vi "translate.vi"(0 "reference":refnum<class "PointNode.lvclass">, 1 "dx":dbl format="%.2f", 2 "dy":dbl format="%.2f", 5 "error in (no error)":errorcluster) -> (14 "reference out":refnum<class "PointNode.lvclass">, 19 "error out":errorcluster)   [LabVIEW 2016, in "PointNode.lvclass"]
doc: "public void translate(double dx, double dy)"
uses:
  <resource>/Framework/Providers/Open_GDS/UML/PointNode_class/PointNode.lvclass
  C:/Program Files (x86)/National Instruments/LabVIEW 2016/resource/Framework/Providers/Open_GDS/UML/AbstractNode_class/AbstractNode.lvclass
  <resource>/Framework/Providers/Open_GDS/UML/General/Point/Point Point2D.ctl
  <resource>/Framework/Providers/Open_GDS/UML/AbstractNode_class/AbstractNode.lvclass
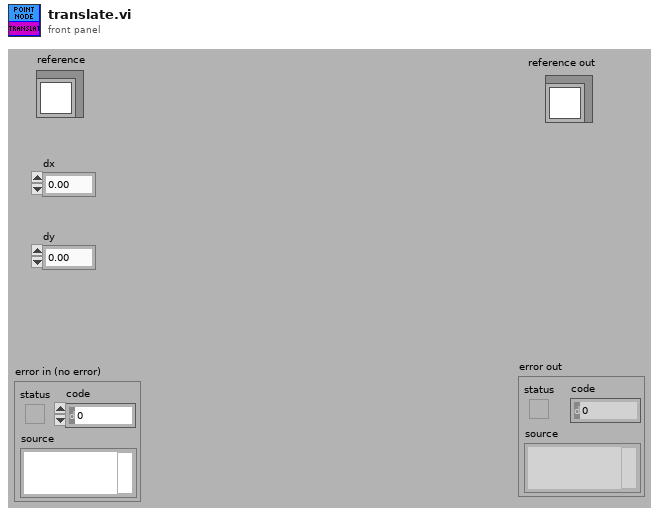
[diagram p1: front panel]
types:
  T1 = typedef "Point Point2D.ctl" = cluster{"x":dbl, "y":dbl}
  T2 = typedef "PointNode.lvclass/ObjectAttributes.ctl" = cluster{"point":T1}
  T3 = typedef "AbstractNode.lvclass/ObjectAttributes.ctl" = cluster{"parent":refnum<class "AbstractNode.lvclass">, "children":refnum<class "AbstractNode.lvclass">[], "Hidden":bool}
  T4 = typedef "Rectangle Rectangle2D.ctl" = cluster{"x":dbl, "y":dbl, "width":dbl, "height":dbl}
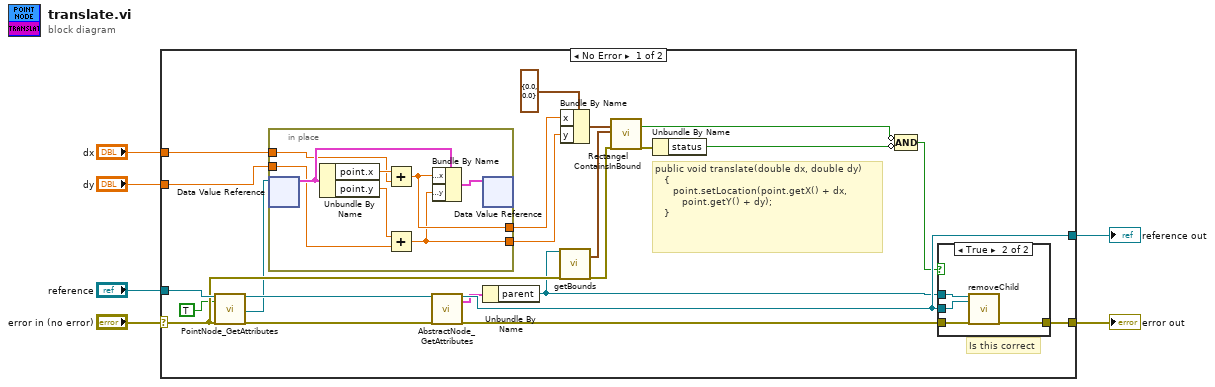
[diagram p0: block diagram]
diagram:
  n1 = case shown="No Error" "error in (no error)" {
    selector: "error in (no error)" -> [w24 w43]
    tunnel: "reference" -> [w29 w44]
    tunnel: [w28 w43] -> w5
    tunnel: [w27 w44] -> w4
    tunnel: "dx" -> [w12 _]
    tunnel: "dy" -> [w11 _]
    frame No Error {
      # "Is this correct"
      # "public void translate(double dx, double dy)\n   {\n      point.setLocation(point.getX() + dx,\n         point.getY() + dy);\n   }"
      n2 = call <resource>:"PointNode_GetAttributes.vi"("reference in"=w29, "OnlyGetDvrReference(False)"=TRUE, "error in (no error)"=w24) -> ("reference out"=w16:refnum<class "PointNode.lvclass">, "DataRef"=w13:refnum<data-value>, "error out"=w15:errorcluster)  [unwired: 13 in, 1 out]
      n3 = in-place {
        in-place-border: w12 -> [w33]
        in-place-border: w11 -> [w32]
        in-place-border: [w31] -> w10
        in-place-border: [w30] -> w9
        n4 = in-place-dvr #1(w13) -> (w37:T2)  [unwired: 1 out]
        n5 = Unbundle By Name(w37) -> ("point.x"=w35:dbl, "point.y"=w34:dbl)
        n6 = Add(x=w35, y=w33) -> (x+y=w31:dbl)
        n7 = Add(x=w34, y=w32) -> (x+y=w30:dbl)
        n8 = Bundle By Name(cluster=w37, "point.x"=w31, "point.y"=w30) -> (w36:T2)
        n9 = in-place-dvr #1(w36) -> ()  [unwired: 2 out]
      }
      n10 = call <resource>:"AbstractNode_GetAttributes.vi"("reference in"=w16, "error in (no error)"=w15) -> ("reference out"=w27:refnum<class "PointNode.lvclass">, "Data"=w8:T3, "error out"=w14:errorcluster)  [unwired: 14 in, 1 out]
      n11 = Unbundle By Name(w8) -> ("parent"=w7:refnum<class "AbstractNode.lvclass">)
      n12 = call-dynamic "getBounds.vi"("reference"=w7, "error in (no error)"=w24) -> ("bounds"=w26:T4, "error out"=w22:errorcluster)  [unwired: 16 out]
      n13 = Bundle By Name(cluster=T1 {"x"=0.0, "y"=0.0} ("point2D"), "x"=w10, "y"=w9) -> (w23:T1)
      n14 = call <resource>:"Rectangel ContainsInBound.vi"("point2D"=w23, "bounds"=w26, "error in (no error)"=w22) -> ("contains"=w19:bool, "error out"=w21:errorcluster)  [unwired: 1 in, 14 out]
      n15 = Unbundle By Name(w21) -> ("status"=w20:bool)
      n16 = Compound Arithmetic op=AND(invert w19, invert w20) -> (w18:bool)
      n17 = case shown="True" w18 {
        tunnel: w7 -> [_ w42]
        tunnel: w27 -> [_ w41]
        tunnel: w14 -> [w38 w40]
        tunnel: [w38 w39] -> w28
        frame False {
        }
        frame True {
          n18 = call-dynamic "removeChild.vi"("reference"=w42, "node"=w41, "error in (no error)"=w40) -> ("error out"=w39:errorcluster)  [unwired: 16 out]
        }
      }
    }
    frame Error {
    }
  }
  "reference out" <- w4
  "error out" <- w5
